vi "DepthProfiling_Proc.vi"(5 "DP_filepath":path=path "", 7 "Params.":variant, 8 "error in (no error)":errorcluster, 9 "Dynamic Params In":refnum<queue>, 10 "Quit_UserEvent":refnum<user-event>, 11 "ControlQueueRef":variant) -> (0 "error out":errorcluster, 2 "Output":variant)   [LabVIEW 2013]
uses:
  Apps_static/ScanParams_SingleLine.ctl
  ProcessMethods/Binning/BinType.ctl
  Files/BinaryHeader.ctl
  ControlDef/QueueRefs.ctl
  ControlDef/LaserCtrl_Method.ctl
  ControlDef/States-AToF.ctl
  <instrlib>/AnalogDiscSDKLv/VIs/DWF_CtrlQueue.ctl
  <instrlib>/AnalogDiscSDKLv/VIs/DWF_State.ctl
  <instrlib>/ESP300/Public/Data/ESP300_State.ctl
  <instrlib>/DG535/Command/DG535_States.ctl
  Hardware/BNC(QuantumComposers)/BNC_States.ctl
  Hardware/FemtoLaser(Legacy)/Laser_Status.ctl
  Hardware/DAQmx(Legacy)/DAQmx_Status.ctl
  ControlDef/Signal.ctl
  ProcessMethods/SignalAverager/ProcessStates.ctl
  Files/WriterState.ctl
  Files/Signal_Segment.ctl
  ControlDef/ProcessingMode.ctl
  Hardware/EPM2000(Legacy)/EPM2K_Status.ctl
  <instrlib>/AnalogDiscSDKLv/VIs/DWF_Signal.ctl
  ControlDef/SampleRateSelector.ctl
  ImagingMS/DirectImaging_State.ctl
  ImagingMS/Imaging_Params.ctl
  ProcessMethods/BioMapConversion/BioMAPWriterCoreParams.ctl
  <vilib>/Utility/error.llb/DialogType.ctl
  <vilib>/Utility/miscctls.llb/LVRowAndColumnTypeDef.ctl
  <vilib>/Analysis/baseanly.llb/Mean (DBL).vi
  UI/Autoscale_Y_Single.vi
  <userlib>/_OpenG.lib/comparison/comparison.llb/I32 Changed__ogtk.vi
  ProcessMethods/Binning/SpectrumBinning.vi
  <instrlib>/ESP300/ESP300.lvlib
  <instrlib>/DG535/SRS_DG535_Lib.lvlib
  <userlib>/Utility/ErrorLog_lib.lvlib
  <vilib>/Analysis/NI_AALBase.lvlib
  <instrlib>/AnalogDiscSDKLv/AnalogDiscSDKLv.lvlib
panel:
  in  "SaveMiddleFile":bool
  out "m/z":dbl=11.0
  out "State":T1(ring)
  in  "Linear/Log":bool
  out "Scan#":i32
  out "PrepScan@Iter 2":i32
  out "PrepScan@Iter":i32
  out "UserEventIter.":i32
  in  "Integration Width (±Da)":dbl=0.5
  in  "m/z (Da)":dbl=11.0
  in  "BinType":T2=enum."ByMass"
  in  "BinWidth":dbl=0.2 min=0.001
  in  "#Layers":i32=1 caption="LayerAverage#" min=1 max=2000 step=1
  in  "Shot#":i32=1 caption="nth of Shot" min=1 max=65535 step=1
  in  "X--":bool
  in  "X++":bool
  in  "Fullscale X":bool
  in  "Fullscale Y":bool
  in  "Y--":bool
  in  "Y++":bool
  out "Depth Profile":dbl[](graph)
  out "Spectra":cluster{"Array":dbl[], dbl[]}(graph)
  in  "Quit":bool
  in  "Cancel":bool
  in  "Peaks of Interest":string[][](table)
  in  "Start":bool
  out "Intensity Graph":dbl[][](graph)
  in  "PeakOI #":i32
  out "MS (Raw)":cluster{"m/z_Array":dbl[], sgl[]}(graph)
  out "Iteration":i32
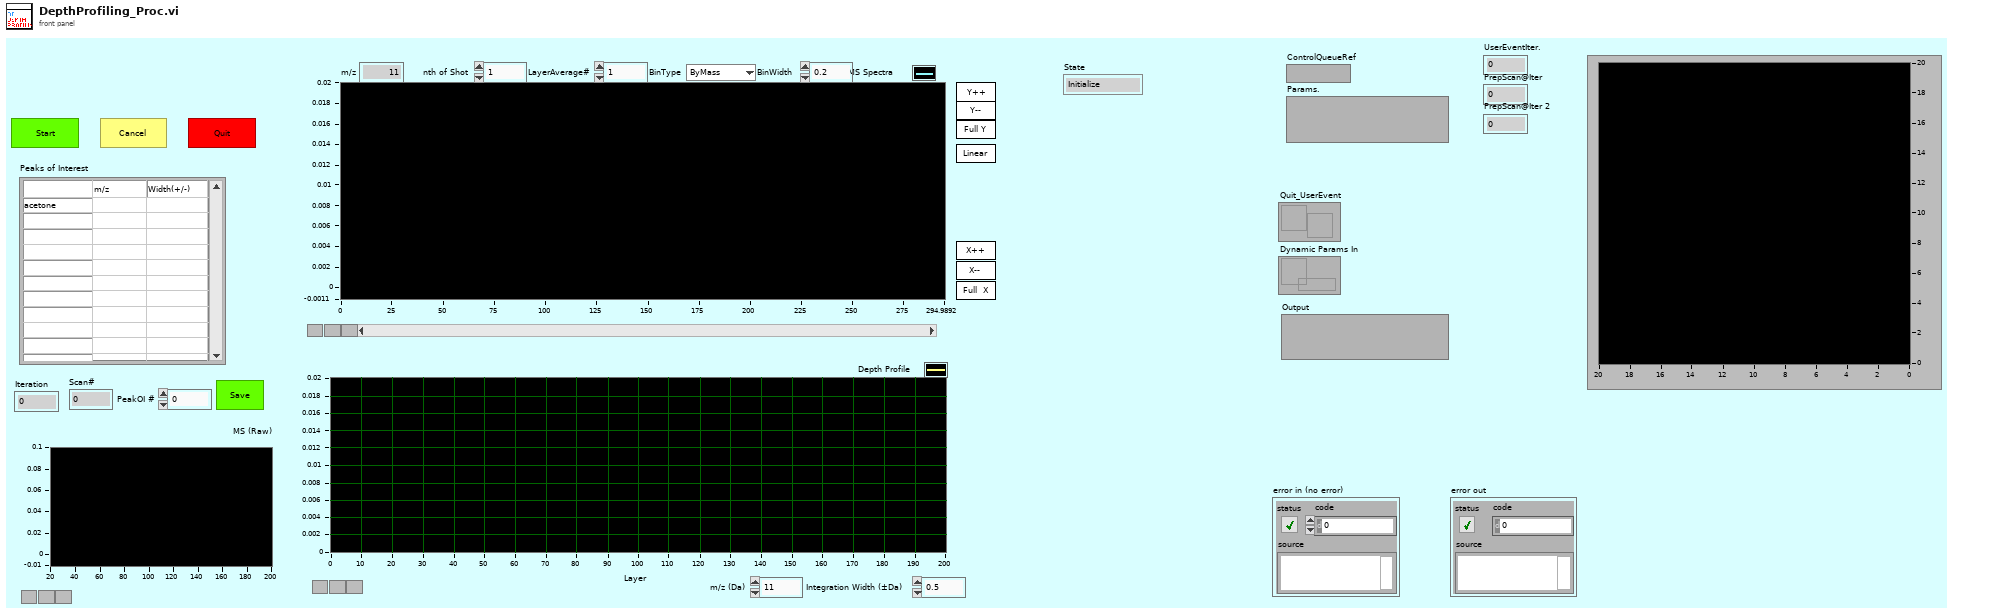
[diagram p1: front panel]
types:
  T1 = enum16{"Initialize", "Open", "PrepScanParams", "WaitData", "Flush", "ScanResult", "CheckEndCondition", "Close", "Quit", "Refresh_Image", "Refresh_Profile", "Refresh_Spectra", "Refresh_RawSpectrum", "SaveMiddleFile", "Save_Image", "SetPeakOI"}
  T2 = typedef "BinType.ctl" = enum16{"ByTime", "ByScreen", "ByMass", "ToUnitMass"}
  T3 = typedef "QueueRefs.ctl" = cluster{"LaserCtrlMethod":T4, "Apps":refnum<queue>, "MainDAQCoreQueue":refnum<queue>, "Micos":refnum<queue>, "ESP300":refnum<queue>, "SMC100":refnum<queue>, "SRS DG535":refnum<queue>, "BNC":refnum<queue>, "SDG_ii":refnum<queue>, "NI-USB_DAQmx":refnum<queue>, "ProcCore_CtrlQueue":refnum<queue>, "WriterCtrl":refnum<queue>, "WriterSIG":refnum<queue>, "Feedback":refnum<queue>, "EPM2000":refnum<queue>, "InfoRef":refnum<vi>, "AppsLock":T5, "ProcCore_SignalQueue":refnum<queue>}
  T4 = typedef "LaserCtrl_Method.ctl" = enum16{"SRS_DG535", "BNC", "SDG_II"}
  T5 = typedef "Semaphore RefNum" = refnum<k1>
  T6 = typedef "ProcessStates.ctl" = enum16{"Initialize", "Normal", "Display", "Write2Buffer", "CalcMzArray", "StartSave", "StopSave", "ConfigChanged", "EndOfLine", "SetFilterParams", "SetGraphsEnable", "SetAcquisitionParams", "ChangeDisplayIncrement", "ChangeRepRate", "SetWriterRef", "Quit", "StartOfLine"}
  T7 = cluster{"Average":i32, "X (Img)":i32, "Y (Img)":i32, "Spectra":sgl[], "Depth":i32, "TickCount":dbl}
  T8 = typedef "BioMAPWriterCoreParams.ctl" = cluster{"File Header":T9, "mzCali.":dbl[], "m/z_Array":dbl[], "SampleRate":T10, "TrigDelay":dbl, "file refnum":refnum<file>, "file path":path, "PeakOI":cluster{"m/z":dbl, "Width(+/-)":dbl}[], "Binning":cluster{"Enable":bool, "BinType":T2, "BinWidth":dbl, "Maximum":dbl, "Minimum":dbl}}
  T9 = typedef "BinaryHeader.ctl" = cluster{"Start Position":dbl[], "StepWidth":dbl[], "Dimension":i32[], "SpecLength":i32}
  T10 = typedef "SampleRateSelector.ctl" = dbl
  T11 = typedef "Imaging_Params.ctl" = cluster{"File Header":T9, "ScanSpeed":dbl, "HighSpeed":dbl, "SampleRate":T10, "Rep.Rate (Hz)":dbl, "TrigDelay":dbl, "mzCali":dbl[], "KeepStill(ms)":u32, "SaveRaw":bool}
  T12 = typedef "DirectImaging_State.ctl" = cluster{"State":enum16{"Initialize", "Open", "PrepScanParams", "WaitData", "Flush", "ScanResult", "CheckEndCondition", "Close", "Quit", "Refresh_Image", "Refresh_Profile", "Refresh_Spectra", "Refresh_RawSpectrum", "SaveMiddleFile", "Save_Image", "SetPeakOI"}, "Para.":variant}
  T13 = cluster{"Save?":bool, "File Header":T9, "Scan#":i32, "ControlRefs":T3, "HighSpeed":dbl, "ScanSpeed":dbl, "SampleRate":T10, "mzCali.":dbl[], "TrigDelay":dbl, "RepRate":dbl, "mzArray":dbl[], "SaveRaw":bool}
  T14 = cluster{"queue out":refnum<queue>, "queue out":refnum<queue>}
  T15 = typedef "Signal.ctl" = cluster{"Command":T6, "Params":variant}
  T16 = typedef "Signal_Segment.ctl" = cluster{"SampleRate":dbl, "TrigDelay":dbl, "SpecLength":dbl, "DAQ_Range":dbl, "Average#":i32, "Position":dbl[], "Spectrum":sgl[], "Calibr.":dbl[], "Pressure":dbl, "Desp_LaserEnergy":dbl, "PI_LaserEnergy":dbl, "Voltages Table":sgl[][], "ProcMode":T17, "Threshold":dbl, "Comment":string, "TickCount":dbl, "Time Stamp":timestamp}
  T17 = typedef "ProcessingMode.ctl" = enum16{"None", "Drop by Threshold", "TDC Simulate", "SetFilter"}
  T18 = typedef "ScanParams_SingleLine.ctl" = cluster{"Start Position":dbl[], "End Position":dbl[], "HighSpeed":dbl, "ScanSpeed":dbl, "KeepStill(ms)":u32, "InstruParams":dbl[]}
  T19 = enum16{"Initialize", "Open", "PrepScanParams", "WaitData", "Flush", "ScanResult", "CheckEndCondition", "Close", "Quit", "Refresh_Image"}
  T20 = cluster{"Average":i32, "X (Img)":i32, "Y (Img)":i32, "Spectra":sgl[], "Depth":i32, "TickCount":dbl}[]
  T21 = typedef "LVRowAndColumnTypeDef.ctl" = cluster{"Row":i32, "Column":i32}
  T22 = typedef "DialogType.ctl" = u16
  T23 = typedef "LVPoint32TypeDef.ctl" = cluster{"Horizontal":i32, "Vertical":i32}
  T24 = typedef "LVRectTypeDef.ctl" = cluster{"Left":i16, "Top":i16, "Right":i16, "Bottom":i16}
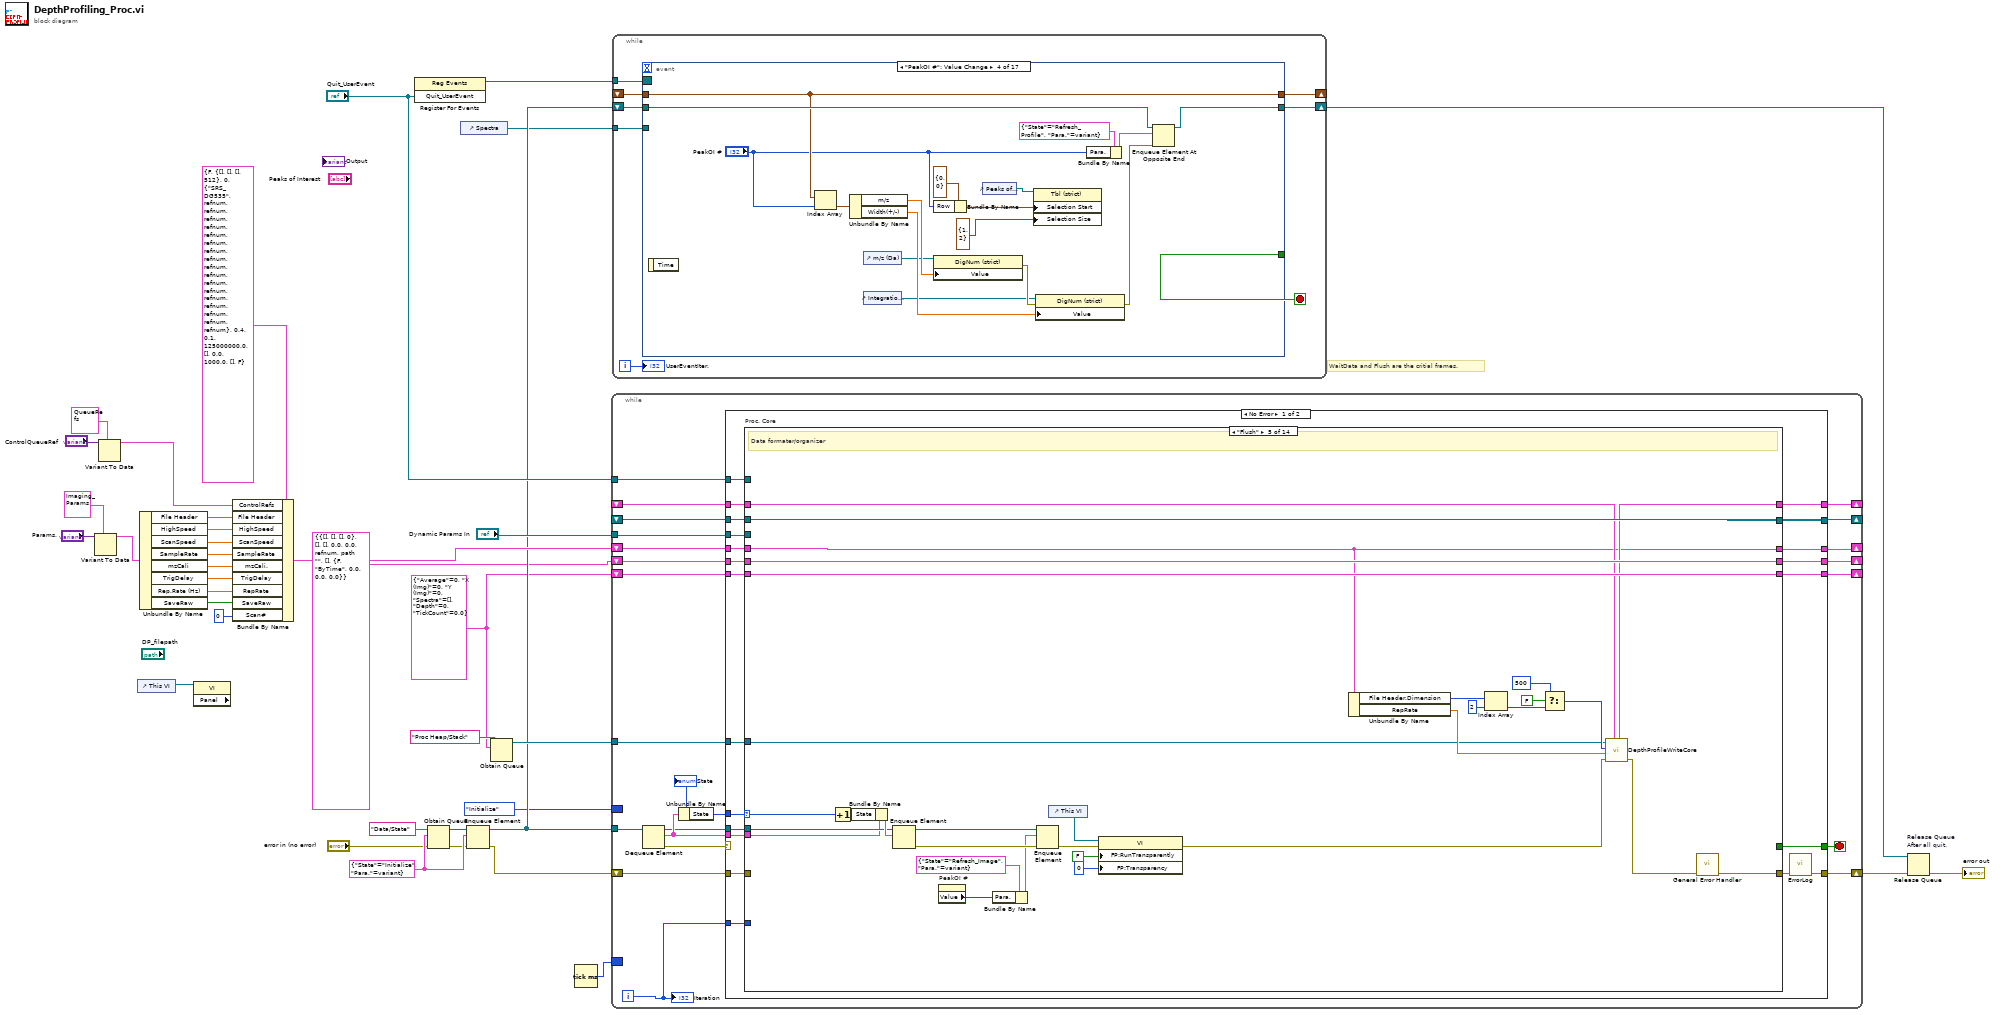
[diagram p0: block diagram]
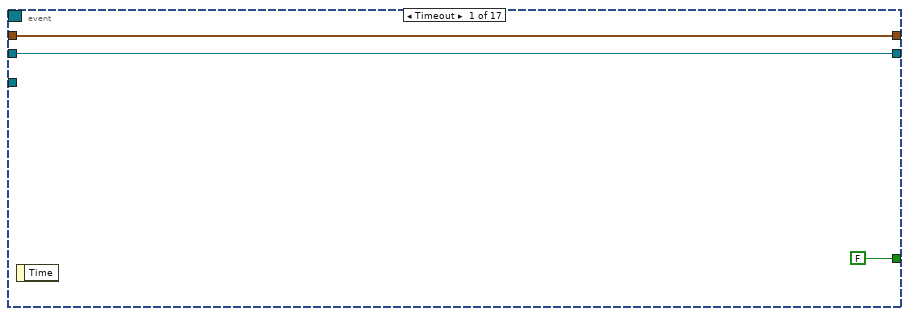
[diagram p2: hidden frame]
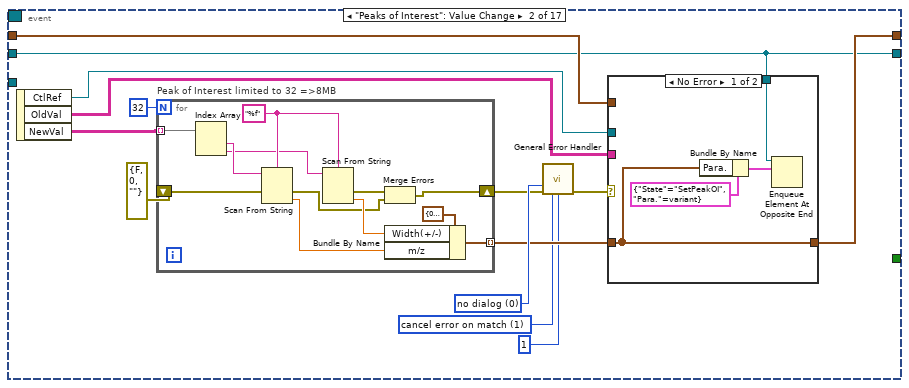
[diagram p3: hidden frame]
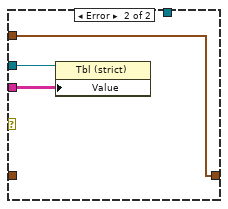
[diagram p4: hidden frame]
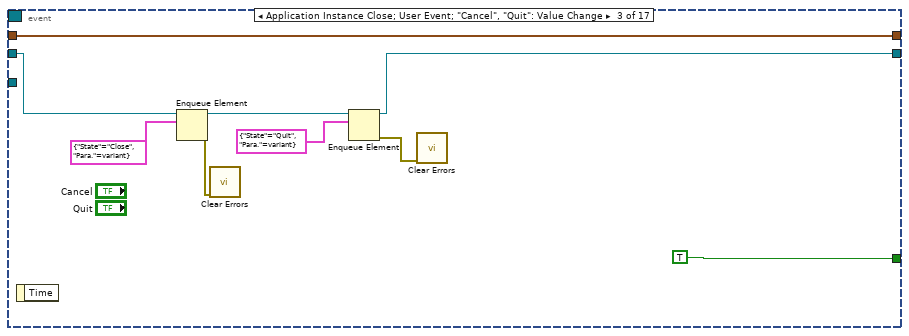
[diagram p5: hidden frame]
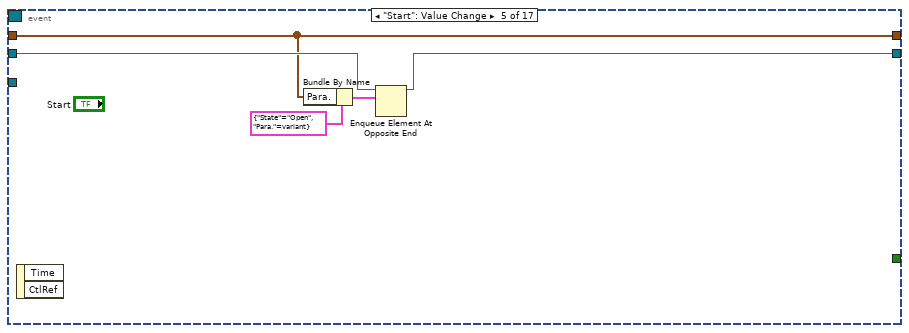
[diagram p6: hidden frame]
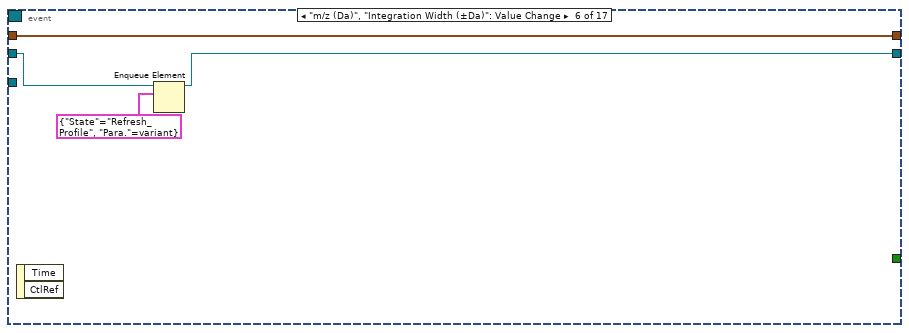
[diagram p7: hidden frame]
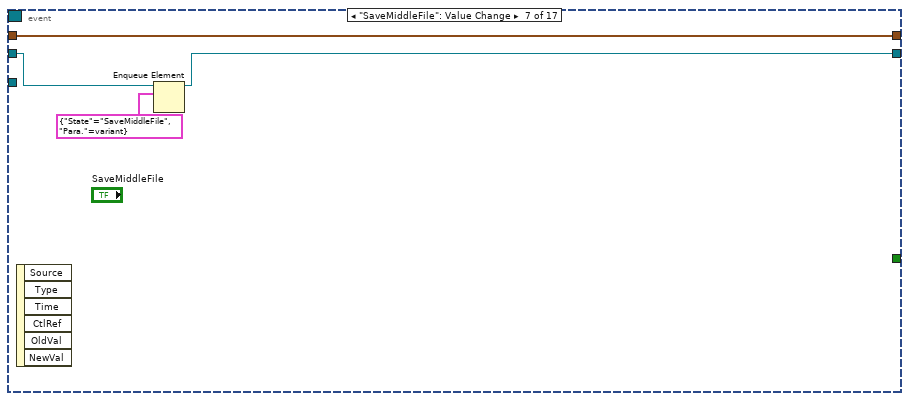
[diagram p8: hidden frame]
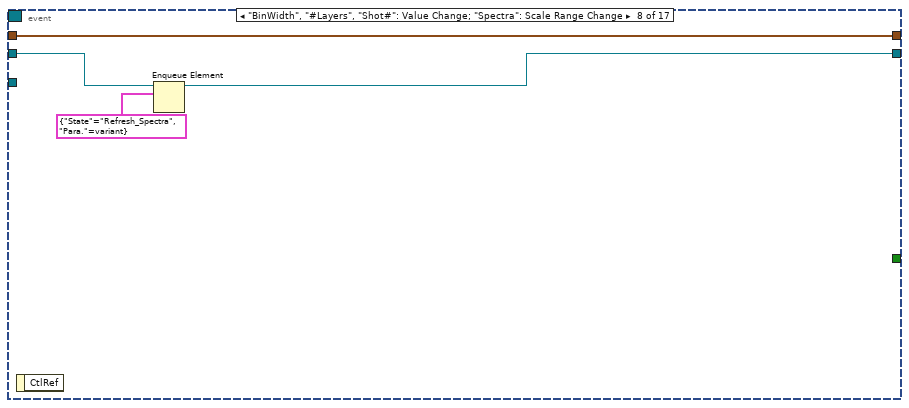
[diagram p9: hidden frame]
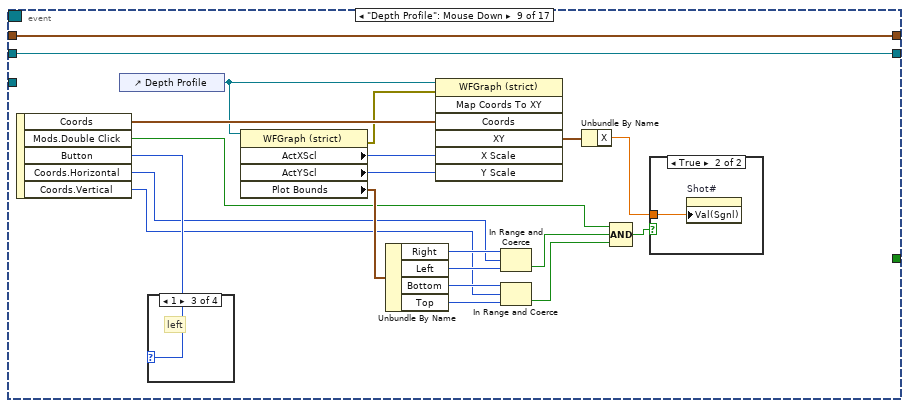
[diagram p10: hidden frame]
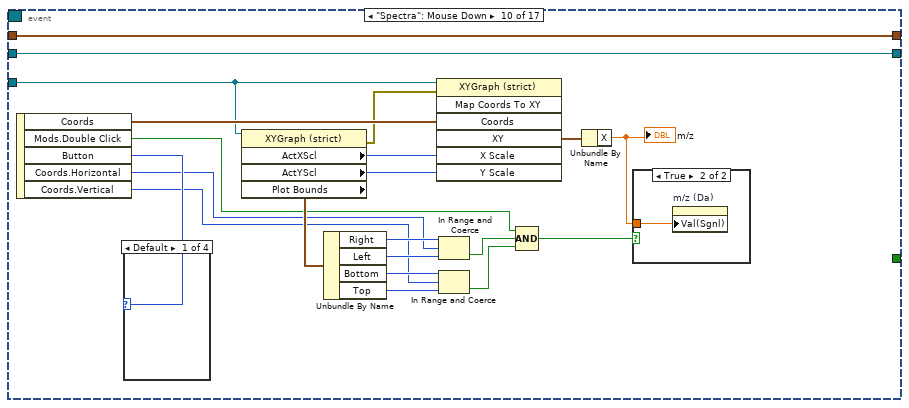
[diagram p15: hidden frame]
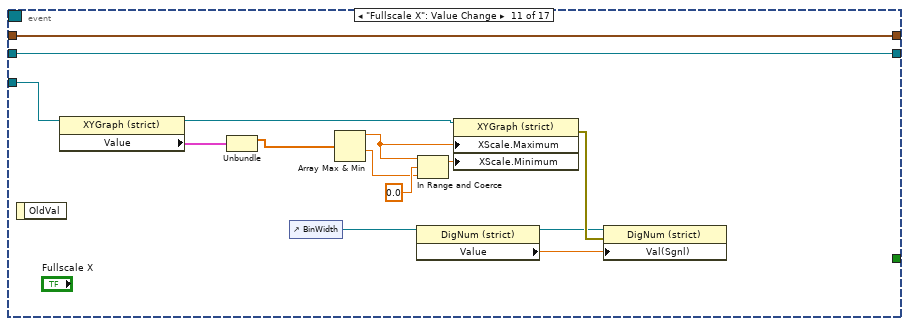
[diagram p20: hidden frame]
diagram:
  w17 = T7 {"Average"=0, "X (Img)"=0, "Y (Img)"=0, "Spectra"=[], "Depth"=0, "TickCount"=0.0} ("output cluster")
  w29 = T12 {"State"=enum."Initialize", "Para."=variant}
  # "WaitData and Flush are the critial frames."
  n1 = Variant To Data(type=T11 {"File Header"={"Start Position"=[], "StepWidth"=[], "Dimension"=[], "SpecLength"=0}, "ScanSpeed"=0.0, "HighSpeed"=0.0, "SampleRate"=0.0, "Rep.Rate (Hz)"=0.0, "TrigDelay"=0.0, "mzCali"=[], "KeepStill(ms)"=0, "SaveRaw"=FALSE} ("BeamProfiling_Params"), Variant="Params.") -> (data=w24:T11)  [unwired: 1 in, 1 out]
  n2 = Variant To Data(type=T3 {"LaserCtrlMethod"=enum."SRS_DG535", "Apps"=refnum, "MainDAQCoreQueue"=refnum, "Micos"=refnum, "ESP300"=refnum, "SMC100"=refnum, "SRS DG535"=refnum, "BNC"=refnum, "SDG_ii"=refnum, "NI-USB_DAQmx"=refnum, "ProcCore_CtrlQueue"=refnum, "WriterCtrl"=refnum, "WriterSIG"=refnum, "Feedback"=refnum, "EPM2000"=refnum, "InfoRef"=refnum, "AppsLock"=refnum, "ProcCore_SignalQueue"=refnum} ("ControlRefs"), Variant="ControlQueueRef") -> (data=w5:T3)  [unwired: 1 in, 1 out]
  n3 = control-ref of="This VI"() -> (w9:refnum<vi>)
  n4 = Unbundle By Name(w24) -> ("File Header"=w23:T9, "HighSpeed"=w22:dbl, "ScanSpeed"=w21:dbl, "SampleRate"=w19:T10, "mzCali"=w11:dbl[], "TrigDelay"=w10:dbl, "Rep.Rate (Hz)"=w2:dbl, "SaveRaw"=w1:bool)
  n5 = property class="VI" props=["Panel"](reference=w9) -> ()  [unwired: 1 in, 3 out]
  n6 = Bundle By Name(cluster=T13 {"Save?"=FALSE, "File Header"={"Start Position"=[], "StepWidth"=[], "Dimension"=[], "SpecLength"=512}, "Scan#"=0, "ControlRefs"={"LaserCtrlMethod"=enum."SRS_DG535", "Apps"=refnum, "MainDAQCoreQueue"=refnum, "Micos"=refnum, "ESP300"=refnum, "SMC100"=refnum, "SRS DG535"=refnum, "BNC"=refnum, "SDG_ii"=refnum, "NI-USB_DAQmx"=refnum, "ProcCore_CtrlQueue"=refnum, "WriterCtrl"=refnum, "WriterSIG"=refnum, "Feedback"=refnum, "EPM2000"=refnum, "InfoRef"=refnum, "AppsLock"=refnum, "ProcCore_SignalQueue"=refnum}, "HighSpeed"=0.4, "ScanSpeed"=0.1, "SampleRate"=125000000.0, "mzCali."=[], "TrigDelay"=0.0, "RepRate"=1000.0, "mzArray"=[], "SaveRaw"=FALSE} ("output cluster"), "ControlRefs"=w5, "File Header"=w23, "HighSpeed"=w22, "ScanSpeed"=w21, "SampleRate"=w19, "mzCali."=w11, "TrigDelay"=w10, "RepRate"=w2, "SaveRaw"=w1, "Scan#"=0) -> (w33:T13)
  n7 = register-events("Quit_UserEvent") -> (reference out=w34:refnum<event-registration>)  [unwired: 2 in, 1 out]
  n8 = Obtain Queue(name (unnamed)="Data/State", element data type=w29, error in (no error)="error in (no error)") -> (queue out=w30:refnum<queue>, error out=w28:errorcluster)  [unwired: 2 in, 1 out]
  n9 = control-ref of="Spectra"() -> (w4:refnum<vi>)
  n10 = Enqueue Element(queue=w30, element=w29, error in (no error)=w28) -> (queue out=w26:refnum<queue>, error out=w18:errorcluster)  [unwired: 1 in, 1 out]
  n11 = Obtain Queue(name (unnamed)="Proc Heap/Stack", element data type=w17) -> (queue out=w38:refnum<queue>)  [unwired: 3 in, 2 out]
  n12 = Tick Count (ms)() -> (millisecond timer value=w16:u32)
  n13 = while {
    shift-right: [w54] -> _
    shift-left: w33 -> [w60]
    tunnel: w26 -> [w59]
    tunnel: w38 -> [w57]
    tunnel: "Dynamic Params In" -> [w51]
    shift-right: [w52] -> _
    shift-left: _ -> [w50]
    shift-right: [w49] -> _
    shift-left: _ -> [w48]
    tunnel: "Quit_UserEvent" -> [w47]
    shift-right: [w45] -> w14
    shift-left: w18 -> [w46]
    shift-right: [w41] -> _
    shift-left: w17 -> [w44]
    shift-right: [w42] -> _
    shift-left: T8 {"File Header"={"Start Position"=[], "StepWidth"=[], "Dimension"=[], "SpecLength"=0}, "mzCali."=[], "m/z_Array"=[], "SampleRate"=0.0, "TrigDelay"=0.0, "file refnum"=refnum, "file path"=path "", "PeakOI"=[], "Binning"={"Enable"=FALSE, "BinType"=enum."ByTime", "BinWidth"=0.0, "Maximum"=0.0, "Minimum"=0.0}} ("output cluster") -> [w43]
    border: w16 -> [_]
    border: ProcessStates."Initialize" -> [_]
    i -> [w39]
    stop <- w53 stop-if-true
    n14 = Dequeue Element(queue=w59) -> (queue out=w55:refnum<queue>, element=w56:T12, error out=w58:errorcluster)  [unwired: 2 in, 1 out]
    n15 = Unbundle By Name(w56) -> ("State"=w40:T1)
    "State" <- w40
    n16 = case shown="No Error" w58 {
      tunnel: w60 -> [w81 w581]
      tunnel: [w80 w581] -> w54
      tunnel: w57 -> [w79 _]
      tunnel: w40 -> [w78 _]
      tunnel: w56 -> [w77 _]
      tunnel: w55 -> [w76 _]
      tunnel: [w75 TRUE] -> w53
      tunnel: [w74 w579] -> w52
      tunnel: w51 -> [w73 _]
      tunnel: w50 -> [w72 w579]
      tunnel: [w71 w578] -> w49
      tunnel: w48 -> [w70 w578]
      tunnel: w47 -> [w69 _]
      tunnel: w46 -> [w68 w577]
      tunnel: [w62 w577] -> w45
      tunnel: w44 -> [w67 w575]
      tunnel: w43 -> [w66 w576]
      tunnel: [w65 w576] -> w42
      tunnel: [w64 w575] -> w41
      tunnel: w39 -> [w61 _]
      frame No Error {
        n17 = case "Proc. Core" shown="\"Flush\"" w78 {
          selector: w78 -> [w85 w163 w233 _ w392 w402 _ _ _ _ _ _ _ _]
          tunnel: w81 -> [w95 w129 w239 w259 w367 w407 w424 w443 w449 w480 w498 w520 w562 w574]
          tunnel: [w95 w170 w230 w259 w367 w407 w424 w443 w449 w480 w498 w520 w562 w574] -> w80
          tunnel: w79 -> [_ _ _ w268 w366 _ _ _ w463 _ _ _ _ _]
          tunnel: w77 -> [w86 w141 w234 w270 w393 w403 w422 _ _ w474 _ _ _ _]
          tunnel: w76 -> [w87 w164 w224 w271 w394 w404 w423 _ _ w481 _ _ _ _]
          tunnel: [_ _ _ _ _ _ _ _ TRUE _ _ _ _ _] -> w75
          tunnel: [w103 w130 w231 w269 w375 w401 w421 w441 w462 w475 w493 w518 w550 w573] -> w74
          tunnel: w73 -> [_ _ w236 _ _ _ _ _ w455 _ _ _ _ _]
          tunnel: w72 -> [w103 _ w231 w269 w378 w401 w421 w441 w462 w475 w493 w518 w550 w573]
          tunnel: [w102 w159 w229 w263 w391 w400 w420 w433 w461 w479 w494 w532 w561 w572] -> w71
          tunnel: w70 -> [w102 _ w229 w263 w391 w400 w420 w433 w461 w479 w494 w532 w561 w572]
          tunnel: w69 -> [_ _ _ _ _ _ _ _ w460 _ _ _ _ _]
          tunnel: w68 -> [w101 w147 w227 w267 _ w399 w418 w432 w451 w478 w506 w531 w548 w571]
          tunnel: [w101 w148 w227 w267 w385 w399 w418 w431 w452 w478 w506 w531 w547 w571] -> w63
          tunnel: w67 -> [w99 w125 w228 w265 w387 w397 w416 _ w454 w476 w504 w529 w560 w569]
          tunnel: w66 -> [w100 w139 w221 w264 w386 w398 w417 w430 w450 w477 w505 w530 w549 w570]
          tunnel: [w97 w150 w221 w264 w386 w398 w417 _ w450 w477 w505 w530 w549 w570] -> w65
          tunnel: [w98 w125 w228 w266 w387 w397 w416 _ w454 w476 w504 w529 w560 w569] -> w64
          tunnel: w61 -> [_ _ w226 _ _ _ _ _ _ _ _ _ _ _]
          frame "Initialize" {
            w88 = cluster{"m/z":dbl, "Width(+/-)":dbl}[] [{"m/z"=110.0, "Width(+/-)"=100.0}]  # 10-210 as default range
            w96 = u32[] [0, 0, 12517567, 12320960, 12189888, 12058817, 11927746, 11731139, 11600067, 9175197, 9044125, 11141318, 11010246, 10813639, 10682568, 10551497, 10354890, 10223818, 10092747, 7930019, 7798948, 9633997, 9502926, 9306319, 9175248, 9044176, 8847569, 8716498, 8585427, 6750377, 6619306, 8126677, 7995606, 7798999, 7667927, 7536856, 7340249, 7209178, 7078106, 5505199, 5374128, 6619357, 6488285, 6291678, 6160607, 6029536, 5832929, 5701857, 5570786, 4325557, 4194486, 5112036, 4980965, 4784358, 4653287, 4522215, 4325608, 4194537, 4063466, 3080380, 3014844, 3604716, 3408109, 3277038, 3277038, 3145966, 3014895, 2818288, 2687217, 2556145, 1900738, 1769666, 2097396, 1900789, 1769717, 1638646, 1507575, 1310968, 1179896, 1048825, 721096, 590024, 590075, 393468, 262397, 131326, 255, 1791, 3327, 4863, 5068, 6348, 9471, 11007, 12543, 14079, 15615, 17151, 18687, 20223, 17612, 18636, 25087, 26623, 28159, 29695, 31231, 32767, 34303, 35839, 29900, 31180, 40447, 41983, 43775, 45311, 46847, 48383, 49919, 51455, 42444, 43724, 56063, 57599, 59135, 60671, 62207, 63743, 65535, 65528, 52418, 52413, 65510, 65504, 65498, 65492, 65486, 65480, 65474, 65468, 52369, 52364, 65449, 65443, 65437, 65431, 65425, 65419, 65413, 65407, 52321, 52316, 65389, 65383, 65377, 65371, 65364, 65358, 65352, 65346, 52272, 52267, 65328, 65322, 65316, 65310, 65304, 65298, 65292, 65286, 52224, 314368, 851712, 1244928, 1638144, 2031360, 2424576, 2817792, 3211008, 3604224, 3197952, 3525632, 4783872, 5177088, 5635840, 6029056, 6422272, 6815488, 7208704, 7601920, 6409216, 6736896, 6736896, 8781568, 9174784, 9568000, 9961216, 10354432, 10747648, 11206400, 11599616, 9554944, 9882624, 12779264, 13172480, 13565696, 13958912, 14352128, 14745344, 15138560, 15531776, 12766208, 13093888, 16776960, 16775170, 16773637, 16771847, 16770314, 16768780, 16766991, 16765457, 13411088, 13409810, 16760601, 16758812, 16757278, 16755745, 16753955, 16752422, 16750888, 16749099, 13398052, 13396774, 16744243, 16742704, 16741166, 16739884, 16738345, 16736807, 16735269, 16733730, 13385753, 13384728, 16729371, 16727833, 16726295, 16725012, 16723474, 16721936, 16720397, 16718859, 13373959, 13372677, 16714500, 16712962, 16777215]  # Color table (Rainbow-striped)
            n18 = disable-structure "Wait for user action" shown="Enabled" {
              disable-tunnel: w87 -> [w106 _]
              disable-tunnel: w86 -> [w105 _]
              disable-tunnel: w85 -> [w104 _]
              frame Disabled {
                n19 = Increment(x=w104) -> (x+1=w107:T1)
                n20 = Bundle By Name(cluster=w105, "State"=w107) -> (w108:T12)
                n21 = Enqueue Element(queue=w106, element=w108) -> ()  [unwired: 2 in, 3 out]
              }
              frame Enabled {
              }
            }
            n22 = Unbundle By Name(w95) -> ("File Header.SpecLength"=w90:i32, "File Header"=w84:T9, "mzCali."=w93:dbl[], "SampleRate"=w91:T10, "TrigDelay"=w92:dbl)
            n23 = Subtract(x=w90, y=64) -> (x-y=w82:i32)
            n24 = in-place "Compensate error in float-point number calculation" {
              n25 = in-place-cluster #1(w84) -> ("StepWidth"=w109:dbl[], "Start Position"=w114:dbl[])
              n26 = Index Array(array=w109) -> (element=w113:dbl)  [unwired: 1 in]
              n27 = Multiply(x=w113, y=0.001) -> (x*y=w111:dbl)
              n28 = in-place {
                in-place-border: w111 -> [w116]
                n29 = in-place-array #2(w114, 0) -> (w117:dbl)
                n30 = Subtract(x=w117, y=w116) -> (x-y=w118:dbl)
                n31 = in-place-array #2(w118) -> (w115:dbl[])  [unwired: 1 out]
              }
              n32 = in-place-cluster #1("StepWidth"=w109, "Start Position"=w115) -> (w83:T9)
            }
            n33 = call "CalcMzArray.vi"("TrigDelay"=w92, "Sample Rate"=w91, "Depth"=w82, "mzCali. (a/b/c)"=w93) -> ("mzArray"=w94:dbl[])  [unwired: 7 in]
            n34 = Bundle By Name(cluster=w100, "File Header.SpecLength"=w82, "m/z_Array"=w94, "File Header"=w83, "mzCali."=w93, "SampleRate"=w91, "TrigDelay"=w92, "PeakOI"=w88) -> (w97:T8)
            n35 = Bundle By Name(cluster=w99, "Depth"=w82) -> (w98:T7)
            n36 = property on="Intensity Graph" class="IntGraph (strict)"("Color Table"=w96) -> ()  [unwired: 2 in, 2 out]
          }
          frame "Open" {
            (unwired) T14 {"queue out"=refnum, "queue out"=refnum} ("output cluster")
            w145 = "ActionCallBack" ("name (unnamed)")
            (unwired) 0
            (unwired) cluster{dbl[], dbl[]}[][] []
            # "8192x32KB*4 = 1GB\n!! attention:\nshould be big"
            n37 = Increment(x=w163) -> (x+1=w165:T1)
            n38 = Unbundle By Name(w129) -> ("File Header.SpecLength"=w119:i32, "File Header.Dimension"=w128:i32[], "mzCali."=w124:dbl[], "SampleRate"=w123:T10, "TrigDelay"=w122:dbl)
            n39 = Unbundle By Name(w139) -> ("PeakOI"=w135:cluster{"m/z":dbl, "Width(+/-)":dbl}[])
            n40 = Unbundle By Name(w141) -> ("Para."=w140:variant)
            n41 = Bundle By Name(cluster=w141, "State"=w165) -> (w166:T12)
            n42 = Variant To Data(type=w135, Variant=w140) -> (data=w137:cluster{"m/z":dbl, "Width(+/-)":dbl}[], error out=w138:errorcluster)  [unwired: 1 in]
            n43 = Enqueue Element(queue=w164, element=w166) -> ()  [unwired: 2 in, 3 out]
            n44 = while {
              tunnel: [w176] -> w149
              tunnel: [w175] -> w151
              tunnel: [w174] -> w148
              tunnel: w147 -> [w173]
              stop <- w177 stop-if-true
              n45 = feedback #3(path "" ("selected path")) -> (w181:path)
              n46 = disable-structure shown="Enabled" {
                disable-tunnel: w181 -> [w190 _]
                disable-tunnel: [w189 _] -> w179
                disable-tunnel: [w188 FALSE ("cancelled")] -> w178
                disable-tunnel: w173 -> [w187 _]
                disable-tunnel: [w186 _] -> w172
                frame Disabled {
                  n47 = Strip Path(path=w190) -> (stripped path=w183:path, name=w184:string)
                  n48 = call "File Dialog2"("start path"=w183, "default name"=w184, "error in"=w187, "pattern (all files)"="*.img", "pattern label"="BioMAP Analyze v7.5") -> ("selected path"=w189:path, "cancelled"=w188:bool, "error out"=w186:errorcluster)  [unwired: 7 in, 1 out]
                }
                frame Enabled {
                }
              }
              n49 = case shown="True" w178 {
                tunnel: w179 -> [w194 _]
                tunnel: [w194 w201] -> w180
                tunnel: w181 -> [_ w201]
                tunnel: [w193 w200] -> w177
                tunnel: [w194 path "" ("selected path")] -> w176
                tunnel: [w193 _] -> w175
                tunnel: [w192 errorcluster {"status"=FALSE, "code"=0, "source"=""} ("error out")] -> w174
                tunnel: w172 -> [w192 _]
                frame False {
                  n50 = Compound Arithmetic op=AND(TRUE) -> (w193:bool)
                }
                frame True {
                  n51 = Two Button Dialog(message="Continue without saving?", 1:"No saving" ("F button name (\"Cancel\")"), 2:"Set Filename" ("T button name (\"OK\")")) -> (T button?=w202:bool)
                  n52 = Not(x=w202) -> (.not. x?=w200:bool)
                }
              }
              n53 = feedback-in #3(w180) -> ()
            }
            n54 = Select(t=w135, s=w138, f=w137) -> (s? t:f=w136:cluster{"m/z":dbl, "Width(+/-)":dbl}[])
            n55 = call "CalcMzArray.vi"("TrigDelay"=w122, "Sample Rate"=w123, "Depth"=w119, "mzCali. (a/b/c)"=w124) -> ("mzArray"=w120:dbl[])  [unwired: 7 in]
            n56 = Initialize Array(sgl 0.0 ("element"), w119) -> (w132:sgl[])
            n57 = Bundle By Name(cluster=w129, "mzArray"=w120) -> (w121:T13)
            n58 = Bundle By Name(cluster=w125, "Spectra"=w132) -> (w133:T7)
            n59 = Index Array(array=w128, index=2) -> (element=w126:i32)
            n60 = Obtain Queue(max queue size (-1, unlimited)=4192, name (unnamed)="BeamProfiling_Buffer", element data type=T16 {"SampleRate"=0.0, "TrigDelay"=0.0, "SpecLength"=0.0, "DAQ_Range"=0.0, "Average#"=0, "Position"=[], "Spectrum"=[], "Calibr."=[], "Pressure"=0.0, "Desp_LaserEnergy"=0.0, "PI_LaserEnergy"=0.0, "Voltages Table"=[], "ProcMode"=enum."None", "Threshold"=0.0, "Comment"="", "TickCount"=0.0, "Time Stamp"=timestamp(0 s since 1904-01-01)} ("Signal Segment")) -> (queue out=w159:refnum<queue>, error out=w158:errorcluster)  [unwired: 2 in, 1 out]
            n61 = Obtain Queue(name (unnamed)=w145, element data type=w145) -> (queue out=w142:refnum<queue>)  [unwired: 3 in, 2 out]
            n62 = Bundle(cluster=T14 {"queue out"=refnum, "queue out"=refnum}, "queue out"=w159, "queue out"=w142) -> (w146:T14)
            n63 = Initialize Array(w133, w126) -> (w130:T20)
            n64 = Unbundle By Name(w121) -> ("ControlRefs.ProcCore_CtrlQueue"=w160:refnum<queue>)
            n65 = Bundle By Name(cluster=T15 {"Command"=enum."SetWriterRef", "Params"=variant} ("element"), "Command"=ProcessStates."SetWriterRef", "Params"=w146) -> (w168:T15)
            n66 = Enqueue Element "Set Data queue"(queue=w160, element=w168, error in (no error)=w158) -> (queue out=w153:refnum<queue>, error out=w144:errorcluster)  [unwired: 1 in, 1 out]
            n67 = Dequeue Element "Wait DataProc Core Ready"(queue=w142, error in (no error)=w144) -> (error out=w143:errorcluster)  [unwired: 1 in, 3 out]
            n68 = Bundle By Name(cluster=T15 {"Command"=enum."SetWriterRef", "Params"=variant} ("element"), "Command"=ProcessStates."StartSave") -> (w155:T15)
            n69 = Enqueue Element "Start Send Data"(queue=w153, element=w155, error in (no error)=w143) -> (error out=w152:errorcluster)  [unwired: 1 in, 2 out]
            n70 = call <vilib>:"Clear Errors.vi"("error in (no error)"=w152) -> ()  [unwired: 6 in, 1 out]
            n71 = Bundle By Name(cluster=w139, "PeakOI"=w136, "file path"=w149) -> (w150:T8)
            n72 = Bundle By Name(cluster=w121, "Save?"=w151) -> (w170:T13)
          }
          frame "PrepScanParams" {
            n73 = Increment(x=w233) -> (x+1=w232:T1)
            n74 = Bundle By Name(cluster=w234, "State"=w232) -> (w223:T12)
            n75 = Unbundle By Name(w239) -> ("Scan#"=w213:i32, "HighSpeed"=w204:dbl, "File Header"=w219:T9, "RepRate"=w216:dbl)  [unwired: 1 out]
            n76 = Increment(x=w213) -> (x+1=w238:i32)
            n77 = Unbundle By Name(w219) -> ("Start Position"=w212:dbl[], "StepWidth"=w208:dbl[], "Dimension"=w218:i32[])
            n78 = Bundle By Name(cluster=w239, "Scan#"=w238) -> (w230:T13)
            n79 = Index Array(array=w218) -> (element #1=w207:i32, element #3=w215:i32)  [unwired: 3 in, 1 out]
            n80 = Quotient & Remainder(x=w213, y=w207) -> (x-y*floor(x/y)=w206:i32, floor(x/y)=w205:i32)
            n81 = Compound Arithmetic op=MULTIPLY(w215, 1000 ("value"), invert w216) -> (w220:dbl)
            n82 = in-place {
              in-place-border: w208 -> [w244]
              in-place-border: w206 -> [w241]
              in-place-border: w205 -> [w240]
              # "Y"
              # "X"
              n83 = in-place-array #4(w212, 0, 1) -> (w249:dbl, w246:dbl)
              n84 = Index Array(array=w244) -> (element #1=w243:dbl, element #2=w242:dbl)  [unwired: 2 in]
              n85 = Multiply(x=w243, y=w241) -> (x*y=w245:dbl)
              n86 = Multiply(x=w242, y=w240) -> (x*y=w248:dbl)
              n87 = Add(x=w249, y=w245) -> (x+y=w250:dbl)
              n88 = Add(x=w246, y=w248) -> (x+y=w247:dbl)
              n89 = in-place-array #4(w250, w247) -> (w211:dbl[])  [unwired: 2 out]
            }
            n90 = Round Toward +Infinity(x=w220) -> (ceil(x): smallest int >= x=w214:dbl)
            n91 = Bundle By Name(cluster=T18 {"Start Position"=[], "End Position"=[], "HighSpeed"=0.0, "ScanSpeed"=0.0, "KeepStill(ms)"=0, "InstruParams"=[]}, "HighSpeed"=w204, "ScanSpeed"=w204, "KeepStill(ms)"=w214, "Start Position"=w211, "End Position"=w211) -> (w235:T18)
            n92 = flat-sequence {
              tunnel: w236 -> [w258]
              tunnel: w235 -> [w257]
              tunnel: w226 -> [w256]
              tunnel: [w256] -> w225
              tunnel: [w253] -> w222
              frame #0 {
                n93 = Enqueue Element "Send scan params"(queue=w258, element=w257, timeout in ms (-1)=1000) -> (timed out?=w253:bool, error out=w254:errorcluster)  [unwired: 1 in, 1 out]
                n94 = call <vilib>:"Clear Errors.vi"("error in (no error)"=w254) -> ()  [unwired: 6 in, 1 out]
              }
            }
            n95 = case shown="False" w222 {
              tunnel: w224 -> [w252 _]
              tunnel: w223 -> [w251 _]
              frame False {
                n96 = Enqueue Element "If not timeout,\ngoto WaitData.\nOtherwise, Idle"(queue=w252, element=w251) -> ()  [unwired: 2 in, 3 out]
              }
              frame True {
              }
            }
            "PrepScan@Iter" <- w226
            "PrepScan@Iter 2" <- w225
          }
          frame "WaitData" {
            # "Data Pre-processor"
            n97 = Dequeue Element "WaitSpectra"(queue=w263, timeout in ms (-1)=1000) -> (element=w262:T16, timed out?=w260:bool)  [unwired: 1 in, 2 out]
            n98 = case shown="True" w260 {
              tunnel: w271 -> [w303 w364]
              tunnel: w270 -> [w302 _]
              tunnel: w268 -> [w301 _]
              tunnel: [w299 w365] -> w266
              tunnel: w265 -> [w298 w365]
              tunnel: w264 -> [w286 _]
              tunnel: w263 -> [w285 _]
              tunnel: w262 -> [w273 _]
              tunnel: w259 -> [w272 _]
              frame False {
                w282 = FALSE  # True for missing EOL (Legacy)
                # "TODO:  Remove average forcing 1 to sum true average#!!"
                n99 = Unbundle By Name(w272) -> ("ControlRefs.WriterSIG"=w274:refnum<queue>)  [unwired: 1 out]
                n100 = Unbundle By Name(w286) -> ("File Header.Start Position"=w289:dbl[], "File Header.StepWidth"=w290:dbl[])
                n101 = Unbundle By Name(w273) -> ("TickCount"=w276:dbl, "Position"=w291:dbl[], "Spectrum"=w280:sgl[], "Average#"=w278:i32, "Comment"=w277:string)
                n102 = String Subset(string=w277, length (rest)=2 ("length (rest)")) -> ()  [unwired: 1 in, 1 out]
                n103 = Type Cast(type=ProcessStates."StartOfLine", x=w277) -> (*(type *) &x=w288:T6)
                n104 = feedback #5() -> (w287:T6)
                n105 = feedback-in #5(w288) -> ()
                n106 = case shown="True" FALSE {
                  tunnel: w273 -> [_ w305]
                  tunnel: w274 -> [_ w304]
                  frame False {
                  }
                  frame True {
                    n107 = Enqueue Element(queue=w304, element=w305) -> ()  [unwired: 2 in, 3 out]
                  }
                }
                n108 = Multiply(x=w280, y=w278) -> (x*y=w279:sgl[])
                n109 = case "Average Spectra in a single pixel" shown="\"EndOfLine\"" w288 {
                  tunnel: w303 -> [w324 w330 w360]
                  tunnel: w301 -> [w323 w328 w358]
                  tunnel: w302 -> [_ w329 w359]
                  tunnel: w298 -> [_ _ w335]
                  tunnel: [_ _ w346] -> w299
                  tunnel: [_ _ w331] -> w292
                  tunnel: w279 -> [_ _ w331]
                  tunnel: w291 -> [_ _ w345]
                  tunnel: w290 -> [_ _ w344]
                  tunnel: w289 -> [_ _ w343]
                  tunnel: w287 -> [_ _ w341]
                  tunnel: [_ _ w336] -> w284
                  tunnel: w278 -> [_ _ w337]
                  tunnel: w276 -> [_ _ w334]
                  frame "EndOfLine" {
                    # "Not idea solution,\nWhy this? Did not I handled this in flush??"
                    # "End of Line"
                    n110 = Get Queue Status(queue=w323) -> (queue out=w322:refnum<queue>, # elements in queue=w321:i32)  [unwired: 2 in, 6 out]
                    n111 = Less?(x=w321, y=5) -> ()  [unwired: 1 out]
                    n112 = case shown="False" FALSE {
                      tunnel: w322 -> [_ w327]
                      tunnel: [T12 {"State"=enum."Flush", "Para."=variant} ("element") T12 {"State"=enum."WaitData", "Para."=variant} ("element")] -> w319
                      frame False {
                      }
                      frame True {
                        n113 = Flush Queue(queue=w327) -> ()  [unwired: 1 in, 3 out]
                      }
                    }
                    n114 = Enqueue Element At Opposite End(queue=w324, element=w319) -> ()  [unwired: 2 in, 3 out]
                  }
                  frame "StartOfLine" {
                    # "New Line"
                    n115 = Enqueue Element "Implied \"WaitData\""(queue=w330, element=w329) -> ()  [unwired: 2 in, 3 out]
                    n116 = Flush Queue(queue=w328) -> ()  [unwired: 1 in, 3 out]
                  }
                  frame Default {
                    # "Normal Spectra"
                    n117 = Index Array(array=w343) -> (element #1=w353:dbl, element #2=w354:dbl)  [unwired: 2 in]
                    n118 = Index Array(array=w344) -> (element #1=w355:dbl, element #2=w356:dbl)  [unwired: 2 in]
                    n119 = Index Array(array=w345) -> (element #1=w340:dbl, element #2=w357:dbl)  [unwired: 2 in]
                    n120 = Enqueue Element "Implied \"WaitData\""(queue=w360, element=w359) -> ()  [unwired: 2 in, 3 out]
                    n121 = Subtract "Y"(x=w357, y=w354) -> (x-y=w350:dbl)
                    n122 = Subtract "X"(x=w340, y=w353) -> (x-y=w351:dbl)
                    n123 = Divide(x=w350, y=w356) -> (x/y=w349:dbl)
                    n124 = Divide(x=w351, y=w355) -> (x/y=w352:dbl)
                    n125 = Round Toward -Infinity(1:w352) -> (0:w347:dbl)
                    n126 = Round Toward -Infinity(1:w349) -> (0:w348:dbl)
                    n127 = To Long Integer(number=w347) -> (32bit integer=w338:i32)
                    n128 = To Long Integer(number=w348) -> (32bit integer=w339:i32)
                    n129 = call-poly <userlib>:"Data Changed__ogtk.vi"("I32"=w339) -> ("Changed"=w336:bool)
                    n130 = call-poly <userlib>:"Data Changed__ogtk.vi"("I32"=w338) -> ("Changed"=w342:bool)
                    n131 = Bundle By Name(cluster=w335, "TickCount"=w334, "X (Img)"=w338, "Y (Img)"=w339, "Spectra"=w331, "Average"=w337) -> (w346:T7)
                    n132 = Or(x=w336, y=w342) -> ()  [unwired: 1 out]
                    n133 = Not Equal?(x=ProcessStates."StartOfLine", y=w341) -> (x != y?=w332:bool)
                    n134 = case shown="True" w332 {
                      tunnel: w358 -> [_ w362]
                      tunnel: w346 -> [_ w361]
                      frame False {
                      }
                      frame True {
                        n135 = Enqueue Element ("Push previous to stack")(queue=w362, element=w361) -> ()  [unwired: 2 in, 3 out]
                      }
                    }
                  }
                }
                n136 = Tick Count (ms)() -> (millisecond timer value=w294:u32)
                n137 = Less?(x=u32 50, y=w294) -> (x < y?=w295:bool)
                n138 = feedback #6() -> (w296:u32)
                n139 = case "raw MS refresh" shown="True" w295 {
                  tunnel: w292 -> [_ w316]
                  tunnel: w294 -> [_ w317]
                  tunnel: [w312 w317] -> w297
                  tunnel: w296 -> [w312 _]
                  tunnel: w286 -> [_ w314]
                  frame False {
                  }
                  frame True {
                    n140 = Unbundle By Name(w314) -> ("m/z_Array"=w315:dbl[])
                    n141 = Bundle("m/z_Array"=w315, w316) -> (→"MS (Raw)":cluster{"m/z_Array":dbl[], sgl[]})  [unwired: 1 in]
                  }
                }
                n142 = feedback-in #6(w297) -> ()
                n143 = And(x=w284, y=w282) -> (x .and. y?=w283:bool)
                n144 = case "For Legacy Format" shown="True" w283 {
                  tunnel: w285 -> [_ w311]
                  frame False {
                  }
                  frame True {
                    n145 = Type Cast(type="", x=ProcessStates."EndOfLine") -> (*(type *) &x=w310:string)
                    n146 = Bundle By Name(cluster=T16 {"SampleRate"=-1.0, "TrigDelay"=0.0, "SpecLength"=0.0, "DAQ_Range"=0.0, "Average#"=0, "Position"=[], "Spectrum"=[], "Calibr."=[], "Pressure"=-1.0, "Desp_LaserEnergy"=-1.0, "PI_LaserEnergy"=-1.0, "Voltages Table"=[], "ProcMode"=enum."None", "Threshold"=-1.0, "Comment"="", "TickCount"=0.0, "Time Stamp"=timestamp(0 s since 1904-01-01)} ("Value"), "Comment"=w310) -> (w306:T16)
                    n147 = Enqueue Element At Opposite End(queue=w311, element=w306) -> ()  [unwired: 2 in, 3 out]
                  }
                }
              }
              frame True {
                # "this frame can be optimized, to minimize unnecessary flushing"
                n148 = Enqueue Element(queue=w364, element=T12 {"State"=enum."Flush", "Para."=variant}) -> ()  [unwired: 2 in, 3 out]
              }
            }
          }
          frame "Flush" {
            # "Data formater/organizer"
            n149 = Increment(x=w392) -> (x+1=w395:T1)
            n150 = Bundle By Name(cluster=w393, "State"=w395) -> (w396:T12)
            n151 = Enqueue Element(queue=w394, element=w396) -> (queue out=w384:refnum<queue>, error out=w382:errorcluster)  [unwired: 2 in, 1 out]
            n152 = property on="PeakOI #" class="DigNum (strict)"() -> ("Value"=w379:i32)  [unwired: 2 in, 2 out]
            n153 = Bundle By Name(cluster=T12 {"State"=enum."Refresh_Image", "Para."=variant} ("element"), "Para."=w379) -> (w380:T12)
            n154 = Enqueue Element(queue=w384, element=w380, error in (no error)=w382) -> (error out=w383:errorcluster)  [unwired: 1 in, 2 out]
            n155 = control-ref of="This VI"() -> (w390:refnum<vi>)
            n156 = property class="VI"(reference=w390, error in=w383, "FP:RunTransparently"=FALSE ("Front Panel Window:Run VI Transparently"), "FP:Transparency"=u8 0 ("Front Panel Window:Transparency")) -> (error out=w377:errorcluster)  [unwired: 1 out]
            n157 = Unbundle By Name(w367) -> ("File Header.Dimension"=w374:i32[], "RepRate"=w372:dbl)
            n158 = Index Array(array=w374, index=2) -> (element=w369:i32)
            n159 = Select(t=500, s=FALSE, f=w369) -> (s? t:f=w368:i32)
            n160 = call "DepthProfileWriteCore.vi"("Buffer In"=w378, "error in"=w377, "RepRate (Hz)"=w372, "Total_Depth (shots)"=w368, "pre-Processed_Buffer"=w366) -> ("error out"=w376:errorcluster, "Buffer Out"=w375:T20)  [unwired: 5 in]
            n161 = call <vilib>:"General Error Handler.vi"("error in (no error)"=w376) -> ("error out"=w385:errorcluster)  [unwired: 10 in, 4 out]
          }
          frame "ScanResult" {
            n162 = Increment(x=w402) -> (x+1=w405:T1)
            n163 = Bundle By Name(cluster=w403, "State"=w405) -> (w406:T12)
            n164 = Enqueue Element(queue=w404, element=w406) -> ()  [unwired: 2 in, 3 out]
          }
          frame "CheckEndCondition" {
            n165 = Unbundle By Name(w424) -> ("Scan#"=w425:i32, "File Header.Dimension"=w426:i32[])
            "Scan#" <- w425
            n166 = Index Array(array=w426) -> (element #1=w411:i32, element #2=w410:i32)  [unwired: 2 in]
            n167 = Increment(x=w425) -> (x+1=w408:i32)
            n168 = Multiply(x=w411, y=w410) -> (x*y=w409:i32)
            n169 = Greater Or Equal? "Determine end condition"(x=w408, y=w409) -> (x >= y?=w412:bool)
            n170 = Select(t=T19."Close" ("State"), s=w412, f=T19."PrepScanParams" ("State")) -> (s? t:f=w413:T19)
            n171 = Bundle By Name(cluster=w422, "State"=w413) -> (w419:T12)
            n172 = Enqueue Element(queue=w423, element=w419) -> ()  [unwired: 2 in, 3 out]
          }
          frame "Close" {
            n173 = Unbundle By Name(w430) -> ("file path"=w427:path)
            n174 = Not Equal?(x=w427, y=path "" ("file path")) -> (x != y?=w429:bool)
            n175 = case shown="True" w429 {
              tunnel: w432 -> [w447 w448]
              tunnel: w430 -> [_ _]
              tunnel: [w447 w448] -> w431
              frame False {
              }
              frame True {
                # "Add write files VIs here"
              }
            }
            n176 = Unbundle By Name(w443) -> ("ControlRefs.ProcCore_CtrlQueue"=w438:refnum<queue>, "ControlRefs.WriterSIG"=w442:refnum<queue>)
            n177 = Bundle By Name(cluster=T15 {"Command"=enum."SetWriterRef", "Params"=variant} ("element"), "Command"=ProcessStates."StopSave") -> (w437:T15)
            n178 = Bundle By Name(cluster=T15 {"Command"=enum."SetWriterRef", "Params"=variant} ("element"), "Command"=ProcessStates."SetWriterRef", "Params"=w442) -> (w445:T15)
            n179 = Enqueue Element(queue=w438, element=w437) -> (queue out=w436:refnum<queue>, error out=w435:errorcluster)  [unwired: 2 in, 1 out]
            n180 = Enqueue Element(queue=w436, element=w445, error in (no error)=w435) -> (error out=w434:errorcluster)  [unwired: 1 in, 2 out]
            n181 = call <vilib>:"Clear Errors.vi"("error in (no error)"=w434) -> ()  [unwired: 6 in, 1 out]
          }
          frame "Quit" {
            n182 = disable-structure shown="Enabled" {
              disable-tunnel: w455 -> [w470 _]
              disable-tunnel: w449 -> [w466 _]
              frame Enabled {
                # "Bad solution: have upper level jump out wait queue"
                n183 = Unbundle By Name(w466) -> ("HighSpeed"=w465:dbl)
                n184 = Bundle By Name(cluster=T18 {"Start Position"=[], "End Position"=[], "HighSpeed"=0.0, "ScanSpeed"=0.0, "KeepStill(ms)"=0, "InstruParams"=[]} ("element"), "HighSpeed"=w465, "ScanSpeed"=w465) -> (w467:T18)
                n185 = Enqueue Element(queue=w470, element=w467) -> (error out=w468:errorcluster)  [unwired: 2 in, 2 out]
                n186 = call <vilib>:"Clear Errors.vi"("error in (no error)"=w468) -> ()  [unwired: 6 in, 1 out]
              }
              frame Disabled {
              }
            }
            n187 = Release Queue(queue=w463, error in (no error)=w451) -> (error out=w453:errorcluster)  [unwired: 1 in, 2 out]
            n188 = Generate User Event(user event=w460, event data cluster=cluster{bool} {TRUE} ("event data")) -> (user event out=w458:refnum<user-event>, error out=w457:errorcluster)  [unwired: 2 in]
            n189 = Destroy User Event(user event=w458, error in=w457) -> (error out=w456:errorcluster)
            n190 = Merge Errors(w456, w453) -> (w452:errorcluster)
          }
          frame "Refresh_Image" {
            # "Call command has to be push to the end not start of the queue."
            n191 = Unbundle By Name(w474) -> ("Para."=w473:variant)
            n192 = Variant To Data(type=1 ("PeakOI #"), Variant=w473) -> (data=w471:i32)  [unwired: 1 in, 1 out]
            n193 = disable-structure shown="Disabled" {
              disable-tunnel: w481 -> [w490 _]
              frame Disabled {
                n194 = Get Queue Status(queue=w490) -> (# pending remove=w489:i32)  [unwired: 2 in, 7 out]
                n195 = Equal To 0?(x=w489) -> (x = 0?=w488:bool)
                n196 = case shown="True" w488 {
                  frame False {
                  }
                  frame True {
                    n197 = One Button Dialog(message="Internal error:\nNothing in queue while refresh curves.") -> ()  [unwired: 1 in, 1 out]
                  }
                }
              }
              frame Enabled {
              }
            }
            n198 = disable-structure shown="Disabled" {
              disable-tunnel: w475 -> [w487 _]
              disable-tunnel: w471 -> [w484 _]
              frame Disabled {
                n199 = Array Subset(array=w487, index (dim 2)=w484, length (dim 2)=1 ("length")) -> (w486:T20)  [unwired: 4 in]
                n200 = Array Size(array=w486) -> ()  [unwired: 1 out]
                n201 = control-ref of="Intensity Graph"() -> (w483:refnum<vi>)
                n202 = property class="IntGraph (strict)" props=["ZScale", "Maximum", "ZScale", "Minimum"](reference=w483, "ZScale.Minimum"=0.0 ("Z Scale.Range:Minimum")) -> ()  [unwired: 2 in, 2 out]
              }
              frame Enabled {
              }
            }
          }
          frame "Refresh_Profile" {
            n203 = Unbundle By Name(w498) -> ("mzArray"=w497:dbl[])
            n204 = Subtract(x="m/z (Da)", y="Integration Width (±Da)") -> (x-y=w502:dbl)
            n205 = Add(x="m/z (Da)", y="Integration Width (±Da)") -> (x+y=w503:dbl)
            n206 = Threshold 1D Array(2:w502, 3:w497) -> (0:w499:dbl)  [unwired: 1 in]
            n207 = Round Toward -Infinity(1:w499) -> (0:w501:dbl)
            n208 = Threshold 1D Array(1:w501, 2:w503, 3:w497) -> (0:w500:dbl)
            n209 = for {
              tunnel: w493 -> [w513] mode=indexing
              tunnel: [w509] -> w492 mode=indexing
              tunnel: w500 -> [w508]
              tunnel: w501 -> [w507]
              n210 = Unbundle By Name(w513) -> ("Spectra"=w512:sgl[])
              n211 = Subtract(x=w508, y=w507) -> (x-y=w511:dbl)
              n212 = Array Subset(array=w512, index=w507, length=w511) -> (w510:sgl[])
              n213 = call-poly <vilib>:"Mean.vi"("X"=w510) -> ("mean"=w509:dbl)  [unwired: 1 out]
            }
            "Depth Profile" <- w492
          }
          frame "Refresh_Spectra" {
            n214 = Decrement(x="Shot#") -> (x-1=w527:i32)
            n215 = for {
              N: "#Layers" -> [_]
              tunnel: w518 -> [w541]
              tunnel: w527 -> [w539]
              shift-right: [w537] -> w523
              shift-left: _ -> [w536]
              tunnel: [w534] -> w525
              tunnel: [w533] -> _ mode=indexing
              i -> [w534]
              n216 = Add(x=w539, y=w534) -> (x+y=w538:i32)
              n217 = Index Array(array=w541, index=w538) -> (element=w540:T7)
              n218 = Unbundle By Name(w540) -> ("Spectra"=w533:sgl[])
              n219 = Equal To 0?(x=w534) -> (x = 0?=w535:bool)
              n220 = case shown="False" w535 {
                tunnel: [w544 w545] -> w537
                tunnel: w536 -> [w543 _]
                tunnel: w533 -> [w542 w545]
                frame False {
                  n221 = Add(x=w542, y=w543) -> (x+y=w544:sgl[])
                }
                frame True {
                }
              }
            }
            n222 = Unbundle By Name(w520) -> ("mzArray"=w519:dbl[])
            n223 = Increment(x=w525) -> (x+1=w526:i32)
            n224 = Reciprocal(x=w526) -> (1/x=w524:dbl)
            n225 = control-ref of="Spectra"() -> (w514:refnum<vi>)
            n226 = Multiply(x=w523, y=w524) -> (x*y=w528:dbl[])
            n227 = call-poly "SpecBinning.vi"("BinType"="BinType", "BinWidth"="BinWidth", "Signal"=w528, "m/z Array"=w519, "GraphRef."=w514) -> ("BinnedSpectrum"=→"Spectra":cluster{"m/z Array":dbl[], "Signal":dbl[]})  [unwired: 5 in, 1 out]
          }
          frame "SaveMiddleFile" {
            n228 = call <vilib>:"Dflt Data Dir.vi"() -> ("App:Default Data Directory"=w546:path)
            n229 = feedback #7(w546) -> (w552:path)
            n230 = Strip Path(path=w552) -> (stripped path=w556:path, name=w555:string)
            n231 = call "File Dialog"("start path"=w556, "default name"=w555, "error in"=w548, "pattern (all files)"="*.dp.bin", "pattern label"="Depth Profile File") -> ("selected path"=w554:path, "cancelled"=w559:bool, "error out"=w551:errorcluster)  [unwired: 7 in, 1 out]
            n232 = case shown="False" w559 {
              tunnel: w554 -> [w566 _]
              tunnel: [w566 w568] -> w553
              tunnel: w552 -> [_ w568]
              tunnel: w551 -> [w565 _]
              tunnel: w550 -> [w567 _]
              tunnel: [w564 _] -> w547
              tunnel: w549 -> [w563 _]
              frame False {
                n233 = call "DepthProfileFormat_Writer.vi"("error in"=w565, "DepthProfilingArray"=w567, "AcquisitionParams."=w563, "depth profile file path"=w566) -> ("error out"=w564:errorcluster)  [unwired: 7 in]
              }
              frame True {
              }
            }
            n234 = feedback-in #7(w553) -> ()
          }
          frame Default {
            # "Doing nothing, if frame not supported by this processing vi"
          }
        }
        n235 = call <userlib>:"ErrorLog.vi"("error in (no error)"=w63) -> ("error out"=w62:errorcluster)  [unwired: 10 in]
      }
      frame Error {
      }
    }
    "Iteration" <- w39
  }
  n236 = while {
    tunnel: w34 -> [w587]
    shift-right: [w586] -> w12
    shift-left: w26 -> [w589]
    shift-right: [w585] -> _
    shift-left: _ -> [w584]
    tunnel: w4 -> [w583]
    i -> [w582]
    stop <- w588 stop-if-true
    n237 = event shown="[3] \"PeakOI #\": Value Change" {
      selector: w587 -> [_ _ _ _ _ _ _ _ _ _ _ _ _ _ _ _ _]
      dyn-events: _ -> [_ _ _ _ _ _ _ _ _ _ _ _ _ _ _ _ _]
      timeout: _ -> [_ _ _ _ _ _ _ _ _ _ _ _ _ _ _ _ _]
      tunnel: w589 -> [w591 w594 w631 w648 w656 w658 w662 w667 w686 w708 w712 w726 w733 w735 w753 w771 w800]
      tunnel: [FALSE _ TRUE _ _ _ _ _ _ _ _ _ _ _ _ _ _] -> w588
      tunnel: [w591 w594 w627 w649 w654 w657 w661 w667 w686 w708 w712 w726 w733 w735 w753 w771 w800] -> w586
      tunnel: [w590 w595 w626 w643 w652 w660 w664 w666 w688 w710 w725 w728 w734 w752 w770 w792 w821] -> w585
      tunnel: w584 -> [w590 w596 w626 w643 w652 w660 w664 w666 w688 w710 w725 w728 w734 w752 w770 w792 w821]
      tunnel: w583 -> [_ _ _ _ _ _ _ _ _ w702 w714 w727 _ w737 w755 w772 w801]
      event Timeout {
        n238 = event-data() -> ()  [unwired: 1 in, 1 out]
      }
      event "Peaks of Interest": Value Change {
        w606 = T22 0 items=["no dialog", "OK message", "continue or stop message", "OK message + warnings", "continue/stop + warnings"] ("type of dialog (OK msg:1)")
        w603 = 1 items=["no exception", "cancel error on match", "set error on match"] ("[exception action] (none:0)")
        n239 = event-data() -> ("CtlRef"=w593:refnum<vi>, "OldVal"=w597:string[][], "NewVal"=w598:string[][])  [unwired: 1 in]
        n240 = for "Peak of Interest limited to 32 =>8MB" {
          N: 32 -> [_]
          tunnel: w598 -> [w618] mode=indexing
          shift-right: [w610] -> w602
          shift-left: errorcluster {"status"=FALSE, "code"=0, "source"=""} ("error IO") -> [w612]
          tunnel: [w611] -> w604 mode=indexing
          w617 = "%f" ("format string")
          n241 = Index Array(array=w618) -> (element #1=w608:string, element #2=w607:string)  [unwired: 2 in]
          n242 = Scan From String(format string=w617, input string=w608, error in=w612) -> (error out=w609:errorcluster, output 1=w614:dbl)  [unwired: 2 in, 2 out]
          n243 = Scan From String(format string=w617, input string=w607) -> (error out=w613:errorcluster, output 1=w615:dbl)  [unwired: 3 in, 2 out]
          n244 = Merge Errors(w613, w609) -> (w610:errorcluster)
          n245 = Bundle By Name(cluster=cluster{"m/z":dbl, "Width(+/-)":dbl} {"m/z"=0.0, "Width(+/-)"=0.0} ("Peak-Of-Interest"), "Width(+/-)"=w615, "m/z"=w614) -> (w611:cluster{"m/z":dbl, "Width(+/-)":dbl})
        }
        n246 = call <vilib>:"General Error Handler.vi"("type of dialog (OK msg:1)"=w606, "error in (no error)"=w602, "[exception action] (none:0)"=w603, "[exception code]"=1) -> ("error out"=w601:errorcluster)  [unwired: 7 in, 4 out]
        n247 = case shown="No Error" w601 {
          tunnel: w597 -> [_ w625]
          tunnel: [w620 w624] -> w595
          tunnel: w604 -> [w620 _]
          tunnel: w596 -> [_ w624]
          tunnel: w594 -> [w619 _]
          tunnel: w593 -> [_ w623]
          frame No Error {
            n248 = Bundle By Name(cluster=T12 {"State"=enum."SetPeakOI", "Para."=variant} ("element"), "Para."=w620) -> (w621:T12)
            n249 = Enqueue Element At Opposite End(queue=w619, element=w621) -> ()  [unwired: 2 in, 3 out]
          }
          frame Error {
            n250 = property on="Property Node" class="Tbl (strict)"(reference=w623, "Value"=w625) -> ()  [unwired: 1 in, 2 out]
          }
        }
      }
      event Application Instance Close; User Event; "Cancel", "Quit": Value Change {
        n251 = event-data() -> ()  [unwired: 1 in, 1 out]
        n252 = Enqueue Element(queue=w631, element=T12 {"State"=enum."Close", "Para."=variant}) -> (queue out=w632:refnum<queue>, error out=w630:errorcluster)  [unwired: 2 in, 1 out]
        n253 = call <vilib>:"Clear Errors.vi"("error in (no error)"=w630) -> ()  [unwired: 6 in, 1 out]
        n254 = Enqueue Element(queue=w632, element=T12 {"State"=enum."Quit", "Para."=variant}) -> (queue out=w627:refnum<queue>, error out=w633:errorcluster)  [unwired: 2 in, 1 out]
        n255 = call <vilib>:"Clear Errors.vi"("error in (no error)"=w633) -> ()  [unwired: 6 in, 1 out]
      }
      event "PeakOI #": Value Change {
        n256 = event-data() -> ()  [unwired: 1 in, 1 out]
        n257 = Index Array(array=w643, index="PeakOI #") -> (element=w641:cluster{"m/z":dbl, "Width(+/-)":dbl})
        n258 = Unbundle By Name(w641) -> ("m/z"=w640:dbl, "Width(+/-)"=w639:dbl)
        n259 = control-ref of="m/z (Da)"() -> (w636:refnum<vi>)
        n260 = control-ref of="Integration Width (±Da)"() -> (w635:refnum<vi>)
        n261 = Bundle By Name(cluster=T21 {"Row"=0, "Column"=0} ("Selection Start"), "Row"="PeakOI #") -> (w646:T21)
        n262 = property class="DigNum (strict)"(reference=w636, "Value"=w640) -> (error out=w638:errorcluster)  [unwired: 1 in, 1 out]
        n263 = control-ref of="Peaks of Interest"() -> (w644:refnum<vi>)
        n264 = property on="Property Node" class="Tbl (strict)"(reference=w644, "Selection Start"=w646, "Selection Size"=T21 {"Row"=1, "Column"=2}) -> ()  [unwired: 1 in, 2 out]
        n265 = property class="DigNum (strict)"(reference=w635, error in=w638, "Value"=w639) -> (error out=w637:errorcluster)  [unwired: 1 out]
        n266 = Bundle By Name(cluster=T12 {"State"=enum."Refresh_Profile", "Para."=variant} ("element"), "Para."="PeakOI #") -> (w650:T12)
        n267 = Enqueue Element At Opposite End(queue=w648, element=w650, error in (no error)=w637) -> (queue out=w649:refnum<queue>)  [unwired: 1 in, 2 out]
      }
      event "Start": Value Change {
        n268 = event-data() -> ()  [unwired: 1 in, 2 out]
        n269 = Bundle By Name(cluster=T12 {"State"=enum."Open", "Para."=variant} ("element"), "Para."=w652) -> (w653:T12)
        n270 = Enqueue Element At Opposite End(queue=w656, element=w653) -> (queue out=w654:refnum<queue>)  [unwired: 2 in, 2 out]
      }
      event "m/z (Da)", "Integration Width (±Da)": Value Change {
        n271 = event-data() -> ()  [unwired: 1 in, 2 out]
        n272 = Enqueue Element(queue=w658, element=T12 {"State"=enum."Refresh_Profile", "Para."=variant}) -> (queue out=w657:refnum<queue>)  [unwired: 2 in, 2 out]
      }
      event "SaveMiddleFile": Value Change {
        n273 = event-data() -> ()  [unwired: 1 in, 6 out]
        n274 = Enqueue Element(queue=w662, element=T12 {"State"=enum."SaveMiddleFile", "Para."=variant}) -> (queue out=w661:refnum<queue>)  [unwired: 2 in, 2 out]
      }
      event "BinWidth", "#Layers", "Shot#": Value Change; "Spectra": Scale Range Change {
        n275 = event-data() -> ()  [unwired: 1 in, 1 out]
        n276 = Enqueue Element(queue=w667, element=T12 {"State"=enum."Refresh_Spectra", "Para."=variant}) -> ()  [unwired: 2 in, 3 out]
      }
      event "Depth Profile": Mouse Down {
        n277 = event-data() -> ("Coords"=w687:T23, "Mods.Double Click"=w670:bool, "Button"=w680:u16, "Coords.Horizontal"=w673:i32, "Coords.Vertical"=w672:i32)  [unwired: 1 in]
        n278 = control-ref of="Depth Profile"() -> (w679:refnum<vi>)
        n279 = case shown="1" w680 {
          frame Default {
          }
          frame 3 {
            # "middle"
          }
          frame 1 {
            # "left"
          }
          frame 2 {
            # "right"
          }
        }
        n280 = property on="Property Node" class="WFGraph (strict)"(reference=w679) -> (error out=w685:errorcluster, "ActXScl"=w682:i32, "ActYScl"=w683:i32, "Plot Bounds"=w678:T24)  [unwired: 1 in, 1 out]
        n281 = Unbundle By Name(w678) -> ("Right"=w677:i16, "Left"=w676:i16, "Bottom"=w675:i16, "Top"=w674:i16)
        n282 = invoke on="Invoke Node" class="WFGraph (strict)" method="Map Coords To XY"(reference=w679, error in=w685, "Coords"=w687, "X Scale"=w682, "Y Scale"=w683) -> ("XY"=w684:cluster{"X":dbl, "Y":dbl})  [unwired: 2 in, 6 out]
        n283 = In Range and Coerce(upper limit=w677, x=w673, lower limit=w676) -> (In Range?=w669:bool)  [unwired: 1 out]
        n284 = In Range and Coerce(upper limit=w675, x=w672, lower limit=w674) -> (In Range?=w668:bool)  [unwired: 1 out]
        n285 = Unbundle By Name(w684) -> ("X"=w681:dbl)
        n286 = Compound Arithmetic op=AND(w670, w669, w668) -> (w671:bool)
        n287 = case shown="True" w671 {
          tunnel: w681 -> [_ w689]
          frame False {
          }
          frame True {
            n288 = property on="Shot#" class="DigNum (strict)"("Val(Sgnl)"=w689) -> ()  [unwired: 2 in, 2 out]
          }
        }
      }
      event "Spectra": Mouse Down {
        n289 = event-data() -> ("Coords"=w709:T23, "Mods.Double Click"=w691:bool, "Button"=w703:u16, "Coords.Horizontal"=w693:i32, "Coords.Vertical"=w692:i32)  [unwired: 1 in]
        n290 = case shown="Default" w703 {
          frame Default {
          }
          frame 3 {
            # "middle"
          }
          frame 1 {
            # "left"
          }
          frame 2 {
            # "right"
          }
        }
        n291 = property on="Property Node" class="XYGraph (strict)"(reference=w702) -> (error out=w707:errorcluster, "ActXScl"=w704:i32, "ActYScl"=w705:i32, "Plot Bounds"=w694:T24)  [unwired: 1 in, 1 out]
        n292 = Unbundle By Name(w694) -> ("Right"=w700:i16, "Left"=w699:i16, "Bottom"=w698:i16, "Top"=w697:i16)
        n293 = invoke on="Invoke Node" class="XYGraph (strict)" method="Map Coords To XY"(reference=w702, error in=w707, "Coords"=w709, "X Scale"=w704, "Y Scale"=w705) -> ("XY"=w706:cluster{"X":dbl, "Y":dbl})  [unwired: 2 in, 6 out]
        n294 = In Range and Coerce(upper limit=w700, x=w693, lower limit=w699) -> (In Range?=w696:bool)  [unwired: 1 out]
        n295 = In Range and Coerce(upper limit=w698, x=w692, lower limit=w697) -> (In Range?=w695:bool)  [unwired: 1 out]
        n296 = Compound Arithmetic op=AND(w691, w696, w695) -> (w690:bool)
        n297 = Unbundle By Name(w706) -> ("X"=w701:dbl)
        "m/z" <- w701
        n298 = case shown="True" w690 {
          tunnel: w701 -> [_ w711]
          frame False {
          }
          frame True {
            n299 = property on="m/z (Da)" class="DigNum (strict)"("Val(Sgnl)"=w711) -> ()  [unwired: 2 in, 2 out]
          }
        }
      }
      event "Fullscale X": Value Change {
        n300 = event-data() -> ()  [unwired: 1 in, 1 out]
        n301 = property class="XYGraph (strict)"(reference=w714) -> (reference out=w721:refnum<vi>, "Value"=w718:cluster{"Array":dbl[], dbl[]})  [unwired: 1 in, 1 out]
        n302 = Unbundle(w718) -> ("Array"=w719:dbl[])  [unwired: 1 out]
        n303 = control-ref of="BinWidth"() -> (w713:refnum<vi>)
        n304 = Array Max & Min(array=w719) -> (max value=w720:dbl, min value=w715:dbl)  [unwired: 2 out]
        n305 = property class="DigNum (strict)"(reference=w713) -> (reference out=w722:refnum<vi>, "Value"=w723:dbl)  [unwired: 1 in, 1 out]
        n306 = In Range and Coerce(upper limit=w720, x=0.0 ("X Scale.Range:Minimum"), lower limit=w715) -> (coerced(x)=w717:dbl)  [unwired: 1 out]
        n307 = property on="Property Node" class="XYGraph (strict)"(reference=w721, "XScale.Maximum"=w720, "XScale.Minimum"=w717) -> (error out=w724:errorcluster)  [unwired: 1 in, 1 out]
        n308 = property class="DigNum (strict)"(reference=w722, error in=w724, "Val(Sgnl)"=w723) -> ()  [unwired: 2 out]
      }
      event "Fullscale Y": Value Change {
        n309 = event-data() -> ()  [unwired: 1 in, 1 out]
        n310 = call-poly "Autoscale_Y.vi"("GraphRef"=w727) -> ()  [unwired: 11 in]
      }
      event "Linear/Log": Value Change {
        n311 = event-data() -> ()  [unwired: 1 in, 1 out]
        n312 = Select(t=u8 1 ("Y Scale.Mapping Mode"), s="Linear/Log", f=u8 0 ("Y Scale.Mapping Mode")) -> (s? t:f=w729:u8)
        n313 = property on="Spectra" class="XYGraph (strict)"("YScale.Mapping Mode"=w729) -> ()  [unwired: 2 in, 2 out]
      }
      event "X++": Value Change {
        n314 = event-data() -> ()  [unwired: 1 in, 1 out]
        n315 = property on="Property Node" class="XYGraph (strict)"(reference=w737) -> (reference out=w748:refnum<vi>, "XScale.Maximum"=w747:dbl, "XScale.Minimum"=w746:dbl)  [unwired: 1 in, 1 out]
        n316 = Add(x=w747, y=w746) -> (x+y=w745:dbl)
        n317 = Subtract(x=w747, y=w746) -> (x-y=w742:dbl)
        n318 = Multiply(x=0.5, y=w745) -> (x*y=w741:dbl)
        n319 = Multiply(x=0.25, y=w742) -> (x*y=w740:dbl)
        n320 = control-ref of="BinWidth"() -> (w736:refnum<vi>)
        n321 = Add(x=w741, y=w740) -> (x+y=w739:dbl)
        n322 = Subtract(x=w741, y=w740) -> (x-y=w738:dbl)
        n323 = property class="DigNum (strict)"(reference=w736) -> (reference out=w749:refnum<vi>, "Value"=w750:dbl)  [unwired: 1 in, 1 out]
        n324 = property on="Property Node" class="XYGraph (strict)"(reference=w748, "XScale.Maximum"=w739, "XScale.Minimum"=w738) -> (error out=w751:errorcluster)  [unwired: 1 in, 1 out]
        n325 = property class="DigNum (strict)"(reference=w749, error in=w751, "Val(Sgnl)"=w750) -> ()  [unwired: 2 out]
      }
      event "X--": Value Change {
        n326 = event-data() -> ()  [unwired: 1 in, 1 out]
        n327 = property on="Property Node" class="XYGraph (strict)"(reference=w755) -> (reference out=w766:refnum<vi>, "XScale.Maximum"=w765:dbl, "XScale.Minimum"=w764:dbl)  [unwired: 1 in, 1 out]
        n328 = control-ref of="BinWidth"() -> (w754:refnum<vi>)
        n329 = Add(x=w765, y=w764) -> (x+y=w763:dbl)
        n330 = Subtract(x=w765, y=w764) -> (x-y=w760:dbl)
        n331 = Multiply(x=0.5, y=w763) -> (x*y=w759:dbl)
        n332 = Multiply(x=1.0, y=w760) -> (x*y=w758:dbl)
        n333 = Add(x=w759, y=w758) -> (x+y=w757:dbl)
        n334 = Subtract(x=w759, y=w758) -> (x-y=w756:dbl)
        n335 = property class="DigNum (strict)"(reference=w754) -> (reference out=w767:refnum<vi>, "Value"=w769:dbl)  [unwired: 1 in, 1 out]
        n336 = property on="Property Node" class="XYGraph (strict)"(reference=w766, "XScale.Maximum"=w757, "XScale.Minimum"=w756) -> (error out=w768:errorcluster)  [unwired: 1 in, 1 out]
        n337 = property class="DigNum (strict)"(reference=w767, error in=w768, "Val(Sgnl)"=w769) -> ()  [unwired: 2 out]
      }
      event "Y--": Value Change {
        n338 = event-data() -> ()  [unwired: 1 in, 1 out]
        n339 = property on="Property Node" class="XYGraph (strict)"(reference=w772) -> (reference out=w791:refnum<vi>, "Value"=w790:cluster{"Array":dbl[], dbl[]}, "XScale.Maximum"=w778:dbl, "XScale.Minimum"=w779:dbl, "YScale.Maximum"=w787:dbl, "YScale.Minimum"=w788:dbl)  [unwired: 1 in, 1 out]
        n340 = Unbundle(w790) -> ("Array"=w776:dbl[], w777:dbl[])
        n341 = for {
          tunnel: w777 -> [w794] mode=indexing
          tunnel: w776 -> [w798] mode=indexing
          tunnel: w779 -> [w797]
          tunnel: w778 -> [w796]
          tunnel: [w793] -> w780 mode=indexing
          n342 = In Range and Coerce(upper limit=w796, x=w798, lower limit=w797) -> (In Range?=w795:bool)  [unwired: 1 out]
          n343 = case shown="True" w795 {
            tunnel: w794 -> [_ w799]
            tunnel: [_ w799] -> w793
            frame False {
              (unwired) nan
            }
            frame True {
            }
          }
        }
        n344 = Array Max & Min(array=w780) -> (min value=w786:dbl)  [unwired: 3 out]
        n345 = In Range and Coerce(upper limit=w787, x=w786, lower limit=w788) -> (coerced(x)=w789:dbl)  [unwired: 1 out]
        n346 = Subtract(x=w787, y=w789) -> (x-y=w781:dbl)
        n347 = Subtract(x=w789, y=w788) -> (x-y=w783:dbl)
        n348 = Multiply(x=2.0, y=w781) -> (x*y=w774:dbl)
        n349 = Multiply(x=2.0, y=w783) -> (x*y=w784:dbl)
        n350 = Add(x=w789, y=w774) -> (x+y=w775:dbl)
        n351 = Subtract(x=w789, y=w784) -> (x-y=w785:dbl)
        n352 = property on="Property Node" class="XYGraph (strict)"(reference=w791, "YScale.Maximum"=w775, "YScale.Minimum"=w785) -> ()  [unwired: 1 in, 2 out]
      }
      event "Y++": Value Change {
        n353 = event-data() -> ()  [unwired: 1 in, 1 out]
        n354 = property on="Property Node" class="XYGraph (strict)"(reference=w801) -> (reference out=w820:refnum<vi>, "Value"=w819:cluster{"Array":dbl[], dbl[]}, "XScale.Maximum"=w807:dbl, "XScale.Minimum"=w808:dbl, "YScale.Maximum"=w816:dbl, "YScale.Minimum"=w817:dbl)  [unwired: 1 in, 1 out]
        n355 = Unbundle(w819) -> ("Array"=w805:dbl[], w806:dbl[])
        n356 = for {
          tunnel: w806 -> [w823] mode=indexing
          tunnel: w805 -> [w827] mode=indexing
          tunnel: w808 -> [w826]
          tunnel: w807 -> [w825]
          tunnel: [w822] -> w809 mode=indexing
          n357 = In Range and Coerce(upper limit=w825, x=w827, lower limit=w826) -> (In Range?=w824:bool)  [unwired: 1 out]
          n358 = case shown="True" w824 {
            tunnel: w823 -> [_ w828]
            tunnel: [_ w828] -> w822
            frame False {
              (unwired) nan
            }
            frame True {
            }
          }
        }
        n359 = Array Max & Min(array=w809) -> (min value=w815:dbl)  [unwired: 3 out]
        n360 = In Range and Coerce(upper limit=w816, x=w815, lower limit=w817) -> (coerced(x)=w818:dbl)  [unwired: 1 out]
        n361 = Subtract(x=w816, y=w818) -> (x-y=w810:dbl)
        n362 = Subtract(x=w818, y=w817) -> (x-y=w812:dbl)
        n363 = Multiply(x=0.5, y=w810) -> (x*y=w803:dbl)
        n364 = Multiply(x=0.5, y=w812) -> (x*y=w813:dbl)
        n365 = Add(x=w818, y=w803) -> (x+y=w804:dbl)
        n366 = Subtract(x=w818, y=w813) -> (x-y=w814:dbl)
        n367 = property on="Property Node" class="XYGraph (strict)"(reference=w820, "YScale.Maximum"=w804, "YScale.Minimum"=w814) -> ()  [unwired: 1 in, 2 out]
      }
    }
    "UserEventIter." <- w582
  }
  n368 = Release Queue "Release Queue\nAfter all quit."(queue=w12, error in (no error)=w14) -> (error out=→"error out":errorcluster)  [unwired: 1 in, 2 out]
